vi "IR Sensor Read.vi"(8 "error in":errorcluster, 10 "Sensor Pin":u8, 11 "Arduino Resource":T1={"VISA resource"="", "Board Type"=enum."Arduino Uno", "Connection Type"=enum."USB / Serial", "Bytes Per Packet (15)"=15}) -> (0 "error out":errorcluster, 2 "MotionDetected":u8, 3 "Arduino Resource":T1={"VISA resource"="", "Board Type"=enum."Arduino Uno", "Connection Type"=enum."USB / Serial", "Bytes Per Packet (15)"=15})   [LabVIEW 2011, in "LabVIEW Interface for Arduino.lvlib"]
doc: "Reads the digital value of the selected Arduino digital input pin (D0 - D13) which the IR Sensor is connected to. The pin must fist be configured as an input using the Arduino Set Digital Pin Mode VI."
uses:
  LabVIEW Interface for Arduino.lvlib
  Private/Type Defs/Arduino Resource.ctl
  Private/Type Defs/Board Type.ctl
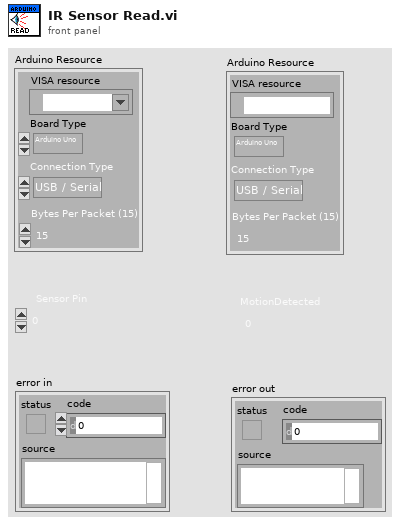
[diagram p1: front panel]
types:
  T1 = typedef "LabVIEW Interface for Arduino.lvlib/Arduino Resource.ctl" = cluster{"VISA resource":refnum<visa-resource-name>, "Board Type":T2, "Connection Type":enum8{"USB / Serial"}, "Bytes Per Packet (15)":u8}
  T2 = typedef "LabVIEW Interface for Arduino.lvlib/Board Type.ctl" = enum16{"Arduino Uno", "Dimuelanove w/Atmega 328", "Mega 2560", "Chipkit Uno32", "Chipkit Max32"}
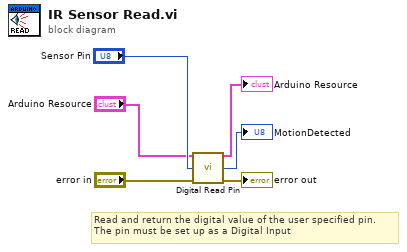
[diagram p0: block diagram]
diagram:
  # "Read and return the digital value of the user specified pin.\nThe pin must be set up as a Digital Input"
  n1 = call "Digital Read Pin.vi"("Arduino Resource"="Arduino Resource", "Digital I/O Pin (0)"="Sensor Pin", "error in"="error in") -> ("Arduino Resource"=→"Arduino Resource":T1, "Value"=→"MotionDetected":u8, "error out"=→"error out":errorcluster)  [unwired: 10 in]
